vi "Seq Motion Data to String.vi"(10 "Motion Data Cluster":T1={"Power Supply Voltage"=0.0, "Min Avg Current"=0.0, "Max Avg Current"=0.0, "Min Run Time"=0.0, "Max Run Time"=0.0, "Min Speed"=0.0, "Max Speed"=0.0, "AP Data % of Threshold"=10.0, "Travel Distance"=0.0, "AP Data Type"=enum."91/61", "Check Current"=FALSE, "Check Run Time"=FALSE, "Check Speed"=FALSE, "Express Motion?"=FALSE, "Check Sound Test"=FALSE, "Check Position?"=FALSE, "Collect AP Data"=FALSE, "Inital Position"=0, "End Position"=0, "Goto Posiition"=0, "Max max Current"=0.0, "Min max Current"=0.0, "Check max Current"=FALSE, "Check Sound"=FALSE, "Min Sound (dB)"=0.0, "Max Sound (dB)"=0.0, "SW Mode"=enum."Hard Switch", "LIN Msg"={"ID"=0, "Msg"=[], "LDF"="EX1H"}} {"LIN Msg"."Msg" format="%02x"; "LIN Msg"."ID" format="%02x"}) -> (2 "Data String":string)   [LabVIEW 2018]
uses:
  type defs/17x Audit Motion Data Seq Control.ctl
  type defs/17x AP Data Type.ctl
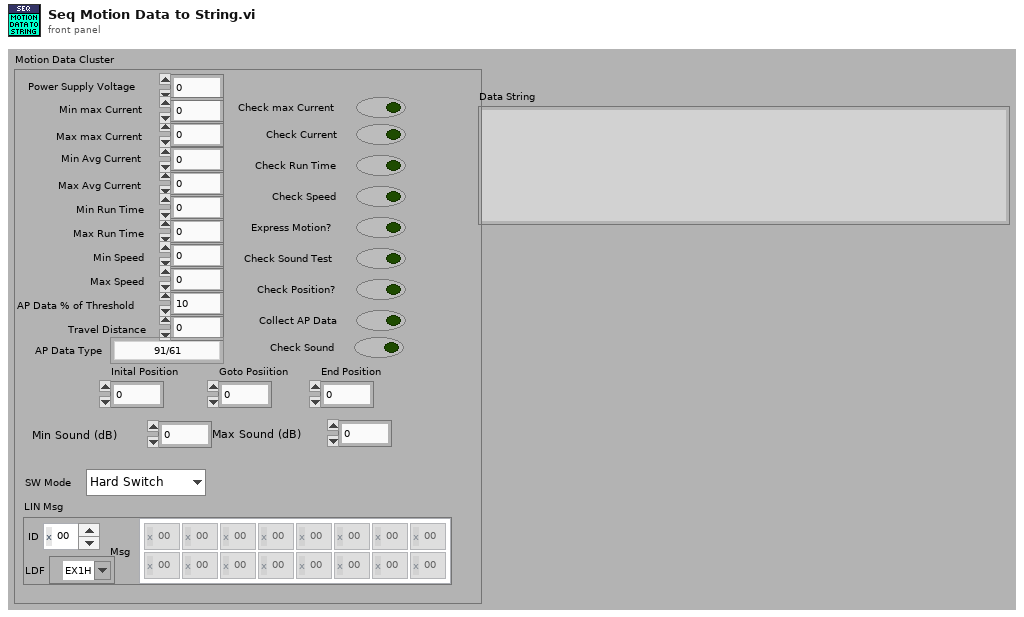
[diagram p1: front panel]
types:
  T1 = typedef "17x Audit Motion Data Seq Control.ctl" = cluster{"Power Supply Voltage":dbl, "Min Avg Current":dbl, "Max Avg Current":dbl, "Min Run Time":dbl, "Max Run Time":dbl, "Min Speed":dbl, "Max Speed":dbl, "AP Data % of Threshold":dbl, "Travel Distance":dbl, "AP Data Type":T2, "Check Current":bool, "Check Run Time":bool, "Check Speed":bool, "Express Motion?":bool, "Check Sound Test":bool, "Check Position?":bool, "Collect AP Data":bool, "Inital Position":u16, "End Position":u16, "Goto Posiition":u16, "Max max Current":dbl, "Min max Current":dbl, "Check max Current":bool, "Check Sound":bool, "Min Sound (dB)":dbl, "Max Sound (dB)":dbl, "SW Mode":enum16{"Hard Switch", "Uncond Frame"}, "LIN Msg":cluster{"ID":u8, "Msg":u8[][], "LDF":refnum<k21>}}
  T2 = typedef "17x AP Data Type.ctl" = enum16{"91/61", "92/62", "93/63", "67", "68", "6F", "71", "91 Msg", "92 Msg", "93 Msg", "94 Msg", "HiRain 91", "HiRain 92 Speed", "HiRain 92 HS", "HiRain 92", "HiRain 93", "SnT"}
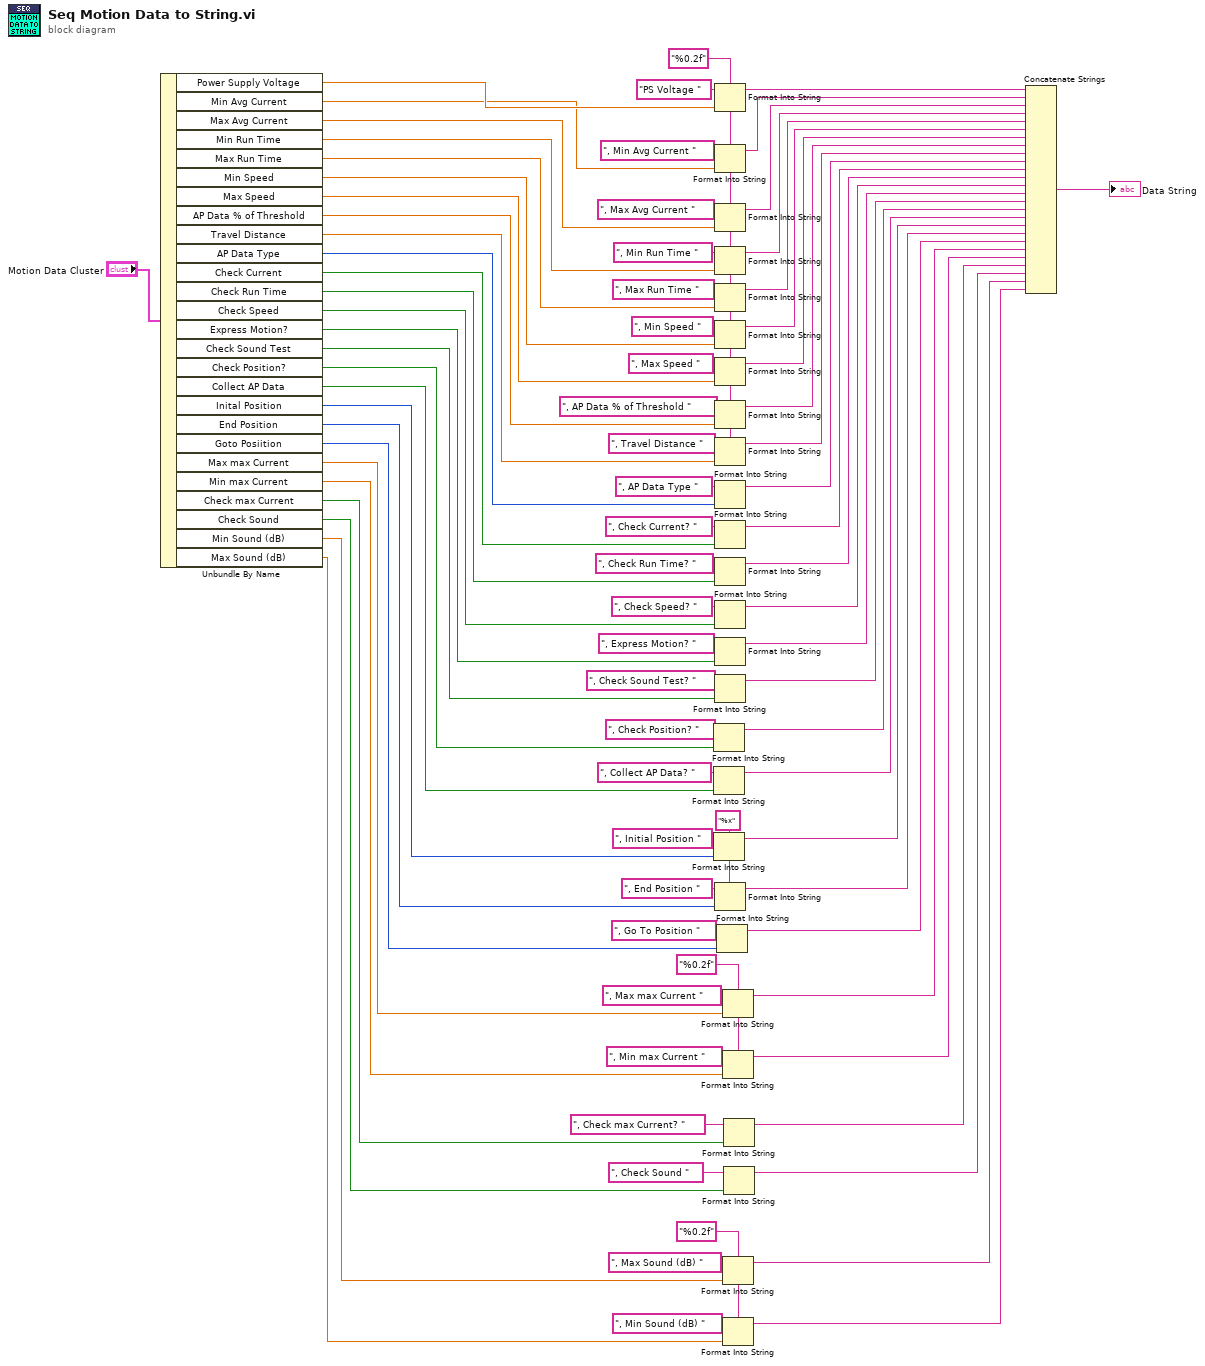
[diagram p0: block diagram]
diagram:
  w6 = "%0.2f" ("format string")
  w20 = "%0.2f" ("format string")
  w32 = "%x" ("format string")
  w21 = "%0.2f" ("format string")
  n1 = Unbundle By Name("Motion Data Cluster") -> ("Power Supply Voltage"=w83:dbl, "Min Avg Current"=w23:dbl, "Max Avg Current"=w80:dbl, "Min Run Time"=w78:dbl, "Max Run Time"=w71:dbl, "Min Speed"=w65:dbl, "Max Speed"=w64:dbl, "AP Data % of Threshold"=w63:dbl, "Travel Distance"=w62:dbl, "AP Data Type"=w61:T2, "Check Current"=w60:bool, "Check Run Time"=w59:bool, "Check Speed"=w58:bool, "Express Motion?"=w57:bool, "Check Sound Test"=w56:bool, "Check Position?"=w38:bool, "Collect AP Data"=w37:bool, "Inital Position"=w31:u16, "End Position"=w30:u16, "Goto Posiition"=w27:u16, "Max max Current"=w17:dbl, "Min max Current"=w16:dbl, "Check max Current"=w15:bool, "Check Sound"=w9:bool, "Min Sound (dB)"=w5:dbl, "Max Sound (dB)"=w4:dbl)
  n2 = Format Into String(initial string=", Check Position? ", w38) -> (resulting string=w36:string)  [unwired: 2 in, 1 out]
  n3 = Format Into String(initial string=", Collect AP Data? ", w37) -> (resulting string=w35:string)  [unwired: 2 in, 1 out]
  n4 = Format Into String(format string=w32, initial string=", Initial Position ", w31) -> (resulting string=w29:string)  [unwired: 1 in, 1 out]
  n5 = Format Into String(format string=w21, initial string="PS Voltage ", w83) -> (resulting string=w55:string)  [unwired: 1 in, 1 out]
  n6 = Format Into String(format string=w21, initial string=", Min Avg Current ", w23) -> (resulting string=w22:string)  [unwired: 1 in, 1 out]
  n7 = Format Into String(format string=w21, initial string=", Max Avg Current ", w80) -> (resulting string=w54:string)  [unwired: 1 in, 1 out]
  n8 = Format Into String(format string=w21, initial string=", Min Run Time ", w78) -> (resulting string=w53:string)  [unwired: 1 in, 1 out]
  n9 = Format Into String(format string=w21, initial string=", Max Run Time ", w71) -> (resulting string=w52:string)  [unwired: 1 in, 1 out]
  n10 = Format Into String(format string=w21, initial string=", Min Speed ", w65) -> (resulting string=w51:string)  [unwired: 1 in, 1 out]
  n11 = Format Into String(format string=w21, initial string=", Max Speed ", w64) -> (resulting string=w50:string)  [unwired: 1 in, 1 out]
  n12 = Format Into String(format string=w21, initial string=", AP Data % of Threshold ", w63) -> (resulting string=w49:string)  [unwired: 1 in, 1 out]
  n13 = Format Into String(format string=w21, initial string=", Travel Distance ", w62) -> (resulting string=w48:string)  [unwired: 1 in, 1 out]
  n14 = Format Into String(initial string=", AP Data Type ", w61) -> (resulting string=w47:string)  [unwired: 2 in, 1 out]
  n15 = Format Into String(initial string=", Check Current? ", w60) -> (resulting string=w46:string)  [unwired: 2 in, 1 out]
  n16 = Format Into String(initial string=", Check Run Time? ", w59) -> (resulting string=w45:string)  [unwired: 2 in, 1 out]
  n17 = Format Into String(initial string=", Check Speed? ", w58) -> (resulting string=w44:string)  [unwired: 2 in, 1 out]
  n18 = Format Into String(initial string=", Express Motion? ", w57) -> (resulting string=w43:string)  [unwired: 2 in, 1 out]
  n19 = Format Into String(initial string=", Check Sound Test? ", w56) -> (resulting string=w42:string)  [unwired: 2 in, 1 out]
  n20 = Format Into String(format string=w32, initial string=", End Position ", w30) -> (resulting string=w28:string)  [unwired: 1 in, 1 out]
  n21 = Format Into String(initial string=", Go To Position ", w27) -> (resulting string=w26:string)  [unwired: 2 in, 1 out]
  n22 = Format Into String(format string=w20, initial string=", Max max Current ", w17) -> (resulting string=w13:string)  [unwired: 1 in, 1 out]
  n23 = Format Into String(format string=w20, initial string=", Min max Current ", w16) -> (resulting string=w12:string)  [unwired: 1 in, 1 out]
  n24 = Format Into String(format string=w6, initial string=", Max Sound (dB) ", w5) -> (resulting string=w2:string)  [unwired: 1 in, 1 out]
  n25 = Format Into String(format string=w6, initial string=", Min Sound (dB) ", w4) -> (resulting string=w1:string)  [unwired: 1 in, 1 out]
  n26 = Format Into String(initial string=", Check max Current? ", w15) -> (resulting string=w11:string)  [unwired: 2 in, 1 out]
  n27 = Format Into String(initial string=", Check Sound ", w9) -> (resulting string=w3:string)  [unwired: 2 in, 1 out]
  n28 = Concatenate Strings(w55, w22, w54, w53, w52, w51, w50, w49, w48, w47, w46, w45, w44, w43, w42, w36, w35, w29, w28, w26, w13, w12, w11, w3, w2, w1) -> (→"Data String":string)
